vi "Subscribe to Roles.vi"(8 "error in (no error)":errorcluster, 9 "Timeout ms (5000)":i32=5000, 10 "SelfQ":refnum<class "MessageQ.lvclass">, 11 "VolatusAPI in":refnum<class "VolatusAPI.lvclass">) -> (0 "error out":errorcluster, 3 "VolatusAPI out":refnum<class "VolatusAPI.lvclass">)   [LabVIEW 2020, in "Volatus.lvlib" / "VolatusAPI.lvclass"]
uses:
  VolatusAPI.lvclass
  VolatusAPI.lvclass/VolatusAPI.ctl
  Role Manager Identity/Role Manager Identity.lvclass
  MessageQ/MessageQ.lvclass
  C:/dev/lv20CE/relink/lv-volatus/Volatus/Role Manager Identity/Role Manager Identity.lvclass
  C:/dev/lv20CE/relink/lv-volatus/Volatus/Identity/Identity.lvclass
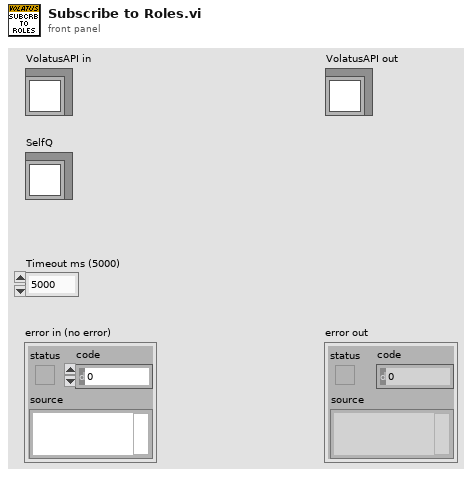
[diagram p1: front panel]
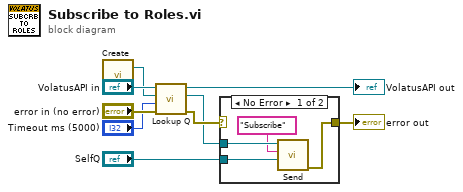
[diagram p0: block diagram]
diagram:
  n1 = call "Create.vi"() -> ("Role Manager Identity out"=w6:refnum<class "Role Manager Identity.lvclass">)  [unwired: 7 in]
  n2 = call "Lookup Q.vi"("error in (no error)"="error in (no error)", "Timeout ms (0)"="Timeout ms (5000)", "Identity"=w6, "VolatusAPI in"="VolatusAPI in") -> ("error out"=w4:errorcluster, "MessageQ"=w3:refnum<class "MessageQ.lvclass">, "VolatusAPI out"=→"VolatusAPI out":refnum<class "VolatusAPI.lvclass">)  [unwired: 5 in]
  n3 = case shown="No Error" w4 {
    selector: w4 -> [_ w14]
    tunnel: w3 -> [w13 _]
    tunnel: "SelfQ" -> [w11 _]
    tunnel: [w10 w14] -> w1
    frame No Error {
      n4 = call "Send.vi"("Data"=w11, "ID"="Subscribe", "MessageQ in"=w13) -> ("error out"=w10:errorcluster)  [unwired: 7 in, 1 out]
    }
    frame Error {
    }
  }
  "error out" <- w1
